vi "TSF Manager Get IMD Settings.vi"(8 "error in (no error)":errorcluster, 11 "TSF Parser in":refnum<class "TSF Parser.lvclass">) -> (0 "error out":errorcluster, 2 "IMD Test Settings out":refnum<class "IMD Test Settings.lvclass">, 3 "TSF Parser out":refnum<class "TSF Parser.lvclass">)   [LabVIEW 2016, in "TSF Parser.lvlib" / "TSF Parser.lvclass"]
uses:
  TSF Parser.lvclass
  Plugins/Test Settings/IMD Test Settings.lvlibp/IMD Test Settings.lvclass
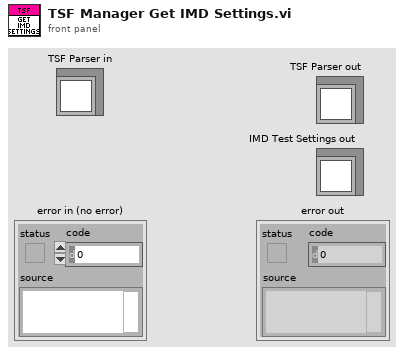
[diagram p1: front panel]
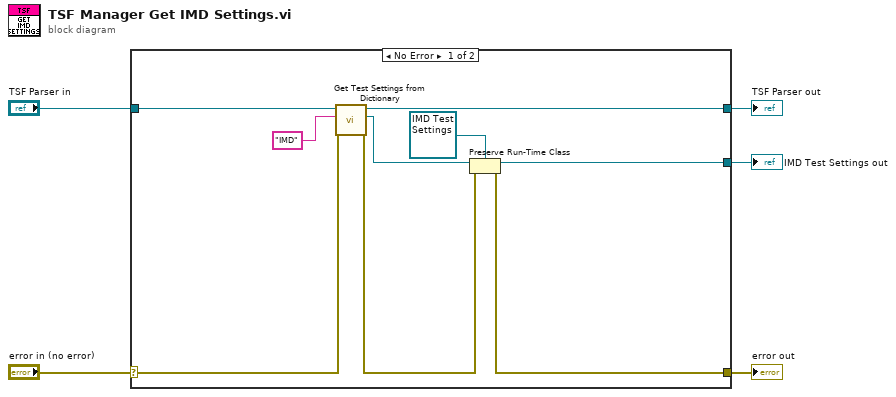
[diagram p0: block diagram]
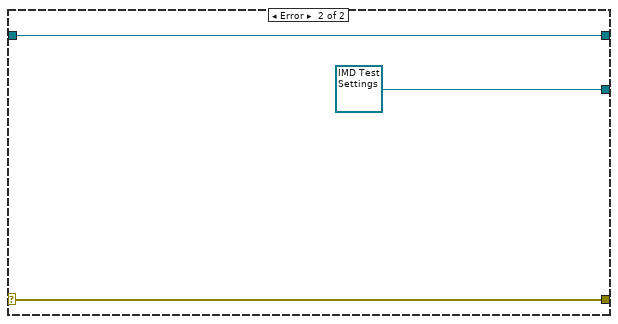
[diagram p2: hidden frame]
diagram:
  n1 = case shown="No Error" "error in (no error)" {
    selector: "error in (no error)" -> [w12 w17]
    tunnel: [w7 w17] -> w4
    tunnel: [w13 w16] -> w2
    tunnel: "TSF Parser in" -> [w14 w16]
    tunnel: [w9 refnum<class "IMD Test Settings.lvclass"> refnum ("IMD Test Settings.lvlibp:IMD Test Settings.lvclass")] -> w1
    frame No Error {
      n2 = call "Get Test Settings from Dictionary.vi"("error in (no error)"=w12, "name"="IMD", "TSF Parser in"=w14) -> ("error out"=w8:errorcluster, "ITestSettings Out"=w10:refnum<class "ITestSettings.lvclass">, "TSF Parser out"=w13:refnum<class "TSF Parser.lvclass">)  [unwired: 6 in]
      n3 = Preserve Run-Time Class(object in=w10, error in=w8, 2:refnum<class "IMD Test Settings.lvclass"> refnum ("IMD Test Settings.lvlibp:IMD Test Settings.lvclass")) -> (object out=w9:refnum<class "IMD Test Settings.lvclass">, error out=w7:errorcluster)
    }
    frame Error {
    }
  }
  "error out" <- w4
  "TSF Parser out" <- w2
  "IMD Test Settings out" <- w1
